vi "Load Config_File Data.vi"(8 "error in (no error)":errorcluster, 9 "Section (\"Default File Data\")":string="Default File Data", 10 "File Data in":T1, 11 "Refnum in":T2) -> (0 "error out":errorcluster, 2 "File Data out":T1, 3 "Refnum out":T2)   [LabVIEW 2019, in "AutoMenuCreator.lvlib"]
uses:
  AutoMenuCreator.lvlib
  Ctl/Ctl_Config_File Data.ctl
  <vilib>/Utility/config.llb/Config Data RefNum.ctl
  <vilib>/Utility/config.llb/NI_LVConfig.lvlib
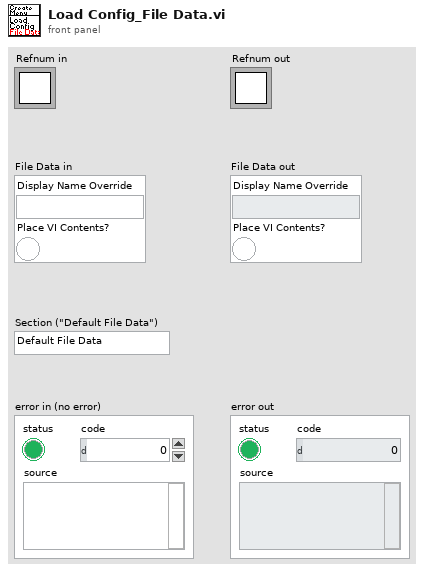
[diagram p1: front panel]
types:
  T1 = typedef "AutoMenuCreator.lvlib/Ctl_Config_File Data.ctl" = cluster{"Display Name Override":string, "Place VI Contents?":bool}
  T2 = typedef "NI_LVConfig.lvlib/Config Data RefNum.ctl" = refnum<k1>
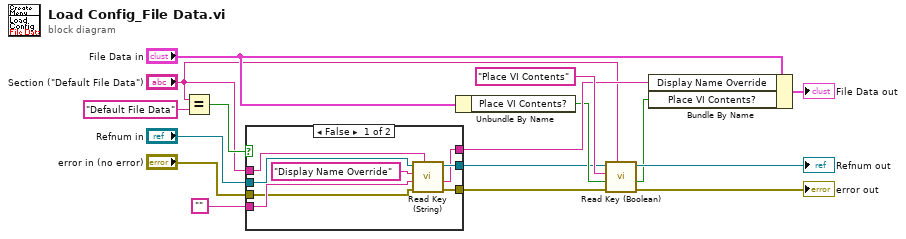
[diagram p0: block diagram]
diagram:
  n1 = Equal?(x="Section (\"Default File Data\")", y="Default File Data") -> (x = y?=w7:bool)
  n2 = case shown="False" w7 {
    tunnel: [w17 w25] -> w12
    tunnel: [w23 w27] -> w5
    tunnel: "Refnum in" -> [w24 w27]
    tunnel: [w18 w26] -> w3
    tunnel: "error in (no error)" -> [w19 w26]
    tunnel: "Section (\"Default File Data\")" -> [w22 _]
    tunnel: "" -> [w20 w25]
    frame False {
      n3 = call <vilib>:"Read Key (String).vi"("section"=w22, "error in (no error)"=w19, "default value"=w20, "key"="Display Name Override", "refnum"=w24) -> ("error out"=w18:errorcluster, "value"=w17:string, "refnum out"=w23:T2)  [unwired: 3 in, 1 out]
    }
    frame True {
    }
  }
  n4 = Unbundle By Name("File Data in") -> ("Place VI Contents?"=w9:bool)
  n5 = call <vilib>:"Read Key (Boolean).vi"("section"="Section (\"Default File Data\")", "error in (no error)"=w3, "default value"=w9, "key"="Place VI Contents", "refnum"=w5) -> ("error out"=→"error out":errorcluster, "value"=w11:bool, "refnum out"=→"Refnum out":T2)  [unwired: 3 in, 1 out]
  n6 = Bundle By Name(cluster="File Data in", "Display Name Override"=w12, "Place VI Contents?"=w11) -> (→"File Data out":T1)
